vi "graph_cluster.vi"() -> ()   [LabVIEW 2020]
uses:
  <vilib>/Analysis/1siggen.llb/Ramp Pattern by Samples.vi
  <vilib>/Analysis/NI_AALBase.lvlib
panel:
  out "graph":cluster{dbl, dbl, "Ramp Pattern":dbl[]}(graph)
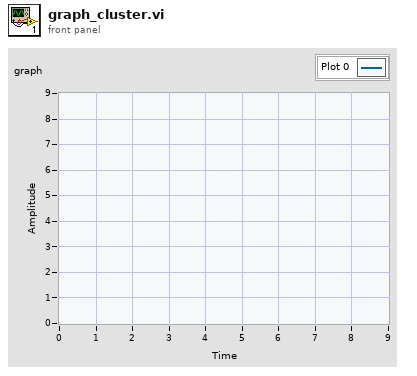
[diagram p1: front panel]
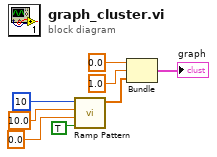
[diagram p0: block diagram]
diagram:
  n1 = call-poly <vilib>:"Ramp Pattern.vi"("exclude end?"=TRUE, "start"=0.0, "end"=10.0, "samples"=10) -> ("Ramp Pattern"=w4:dbl[])  [unwired: 6 in, 1 out]
  n2 = Bundle(0.0, 1.0, "Ramp Pattern"=w4) -> (→"graph":cluster{dbl, dbl, "Ramp Pattern":dbl[]})  [unwired: 1 in]
